vi "fgt get sensor Value.vi"(8 "error in (no error)":errorcluster, 11 "sensorIndex":u32) -> (0 "error out":errorcluster, 3 "value out":sgl)   [LabVIEW 2020, in "fgt_SDK.lvlib"]
doc: "Read sensor value in selected unit, default is \"µl/min\" for flowrate sensors and 'mbar' for pressure sensors"
uses:
  fgt_SDK.lvlib
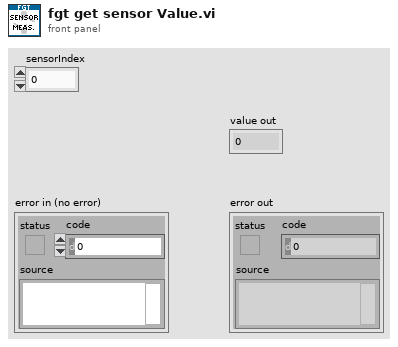
[diagram p1: front panel]
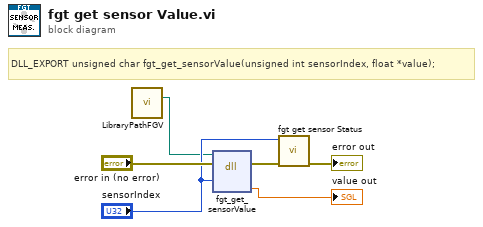
[diagram p0: block diagram]
diagram:
  # "DLL_EXPORT unsigned char fgt_get_sensorValue(unsigned int sensorIndex, float *value);"
  n1 = call "LibraryPathFGV.vi"() -> ("Path Out"=w1:path)  [unwired: 14 in, 1 out]
  n2 = dll-call lib="C:/Workspace/fgt-SDK/LabVIEW/dlls/fgt_SDK_*.*" fn="fgt_get_sensorValue"(path in=w1, error in="error in (no error)", "sensorIndex"="sensorIndex") -> (error out=w4:errorcluster, "value"=→"value out":sgl)  [unwired: 4 in, 1 out]
  n3 = call "fgt get sensor Status.vi"("error in (no error)"=w4, "pressureIndex"="sensorIndex") -> ("error out"=→"error out":errorcluster)  [unwired: 9 in]
